vi "PV Factory Test Mode Data.vi"(11 "result string":string) -> (3 "Boolean":bool)   [LabVIEW 2023]
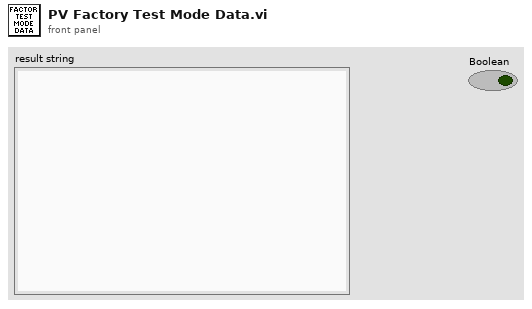
[diagram p1: front panel]
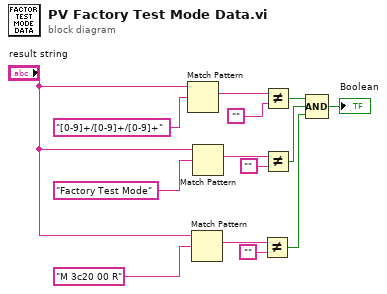
[diagram p0: block diagram]
diagram:
  n1 = Match Pattern(string="result string", regular expression="[0-9]+/[0-9]+/[0-9]+" ("string")) -> (match substring=w13:string)  [unwired: 1 in, 3 out]
  n2 = Match Pattern(string="result string", regular expression="M 3c20 00 R" ("string")) -> (match substring=w11:string)  [unwired: 1 in, 3 out]
  n3 = Match Pattern(string="result string", regular expression="Factory Test Mode" ("string")) -> (match substring=w5:string)  [unwired: 1 in, 3 out]
  n4 = Not Equal?(x=w11, y="") -> (x != y?=w12:bool)
  n5 = Not Equal?(x=w13, y="") -> (x != y?=w6:bool)
  n6 = Not Equal?(x=w5, y="") -> (x != y?=w7:bool)
  n7 = Compound Arithmetic op=AND(w6, w7, w12) -> (→"Boolean":bool)
